vi "Database.GetThisStatus.vi"(7 "system":string, 8 "error in":errorcluster, 9 "Serial":string, 10 "Variant":string, 11 "Data in":T1 {"Variant"."TS"."TV"."minimum" format="%#.3f"; "Variant"."TS"."TV"."maximum" format="%#.3f"; "Variant"."TS"."TP"."value" format="%#.3f"}) -> (0 "error out":errorcluster, 1 "Repetitions":u8, 2 "Status":i8, 3 "Data out":T1 {"Variant"."TS"."TV"."minimum" format="%#.3f"; "Variant"."TS"."TV"."maximum" format="%#.3f"; "Variant"."TS"."TP"."value" format="%#.3f"})   [LabVIEW 2016]
uses:
  Database.Main.Data.ctl
  Database.Main.Data.Status.ctl
  Database.Main.Data.Sets.ctl
  Database.Main.Data.Results.ctl
  ProdaNG/Controls/ProdaNG.Identification.ctl
  ProdaNG/Controls/ProdaNG.ProcessResult.ctl
  ProdaNG/Controls/ProdaNG.ProcessStepResult.ctl
  ProdaNG/Controls/ProdaNG.TestStepResult.ctl
  ProdaNG/Controls/ProdaNG.TestValueResult.ctl
  Database.Main.Data.Variant.ctl
  ProdaNG/Controls/ProdaNG.ProcessStepParam.ctl
  ProdaNG/Controls/ProdaNG.TestStep.ctl
  ProdaNG/Controls/ProdaNG.TestStepParam.ctl
  ProdaNG/Controls/ProdaNG.TestValue.ctl
  tools/EventLog/EventLog.EventLevel.ctl
  tools/EventLog/EventLog.EventSource.ctl
  tools/Translator/Translator.Message.ctl
  tools/EventLog/EventLog.New(array).vi
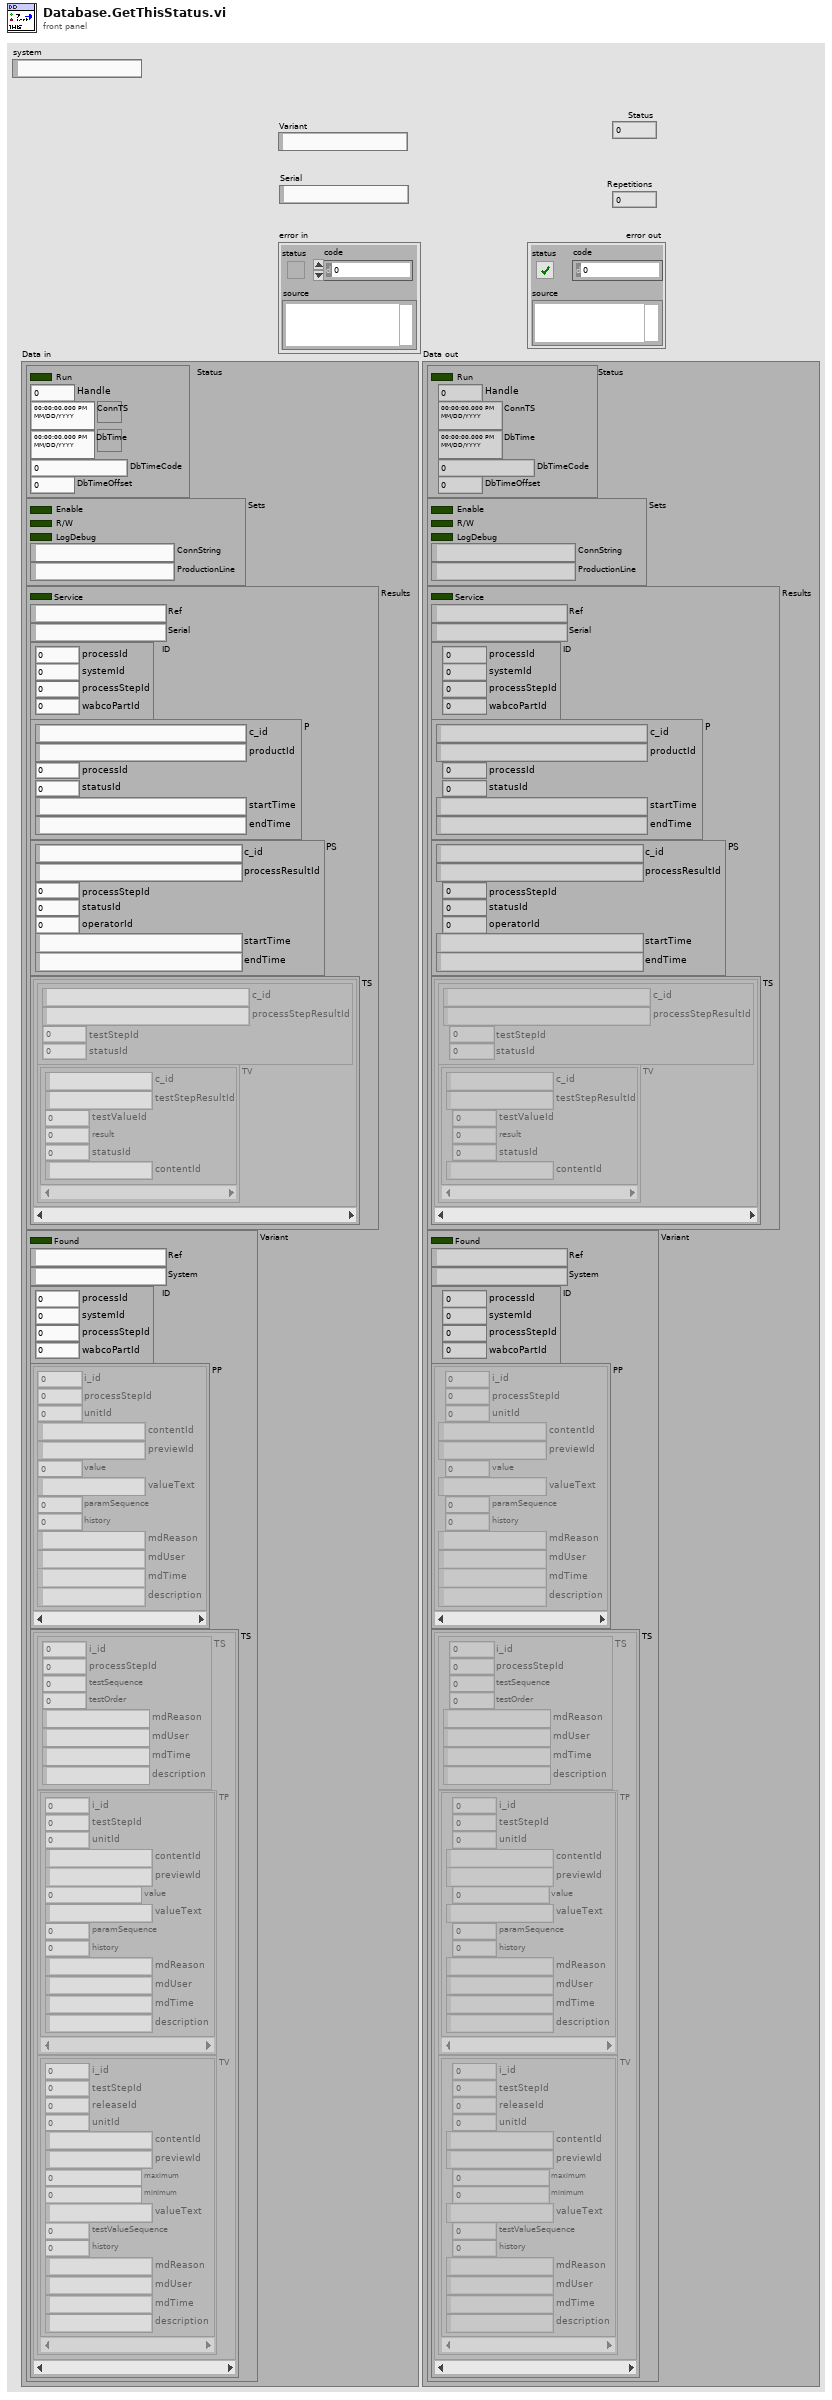
[diagram p1: front panel]
types:
  T1 = typedef "Database.Main.Data.ctl" = cluster{"Status":T2, "Sets":T3, "Results":T4, "Variant":T10}
  T2 = typedef "Database.Main.Data.Status.ctl" = cluster{"Run":bool, "Handle":i32, "ConnTS":timestamp, "DbTime":timestamp, "DbTimeCode":dbl, "DbTimeOffset":dbl}
  T3 = typedef "Database.Main.Data.Sets.ctl" = cluster{"Enable":bool, "R/W":bool, "LogDebug":bool, "ConnString":string, "ProductionLine":string}
  T4 = typedef "Database.Main.Data.Results.ctl" = cluster{"Service":bool, "Ref":string, "Serial":string, "ID":T5, "P":T6, "PS":T7, "TS":cluster{"TS":T8, "TV":T9[]}[]}
  T5 = typedef "ProdaNG.Identification.ctl" = cluster{"processId":i32, "systemId":i32, "processStepId":i32, "wabcoPartId":i32}
  T6 = typedef "ProdaNG.ProcessResult.ctl" = cluster{"c_id":string, "productId":string, "processId":i32, "statusId":i32, "startTime":string, "endTime":string}
  T7 = typedef "ProdaNG.ProcessStepResult.ctl" = cluster{"c_id":string, "processResultId":string, "processStepId":i32, "statusId":i32, "operatorId":i32, "startTime":string, "endTime":string}
  T8 = typedef "ProdaNG.TestStepResult.ctl" = cluster{"c_id":string, "processStepResultId":string, "testStepId":i32, "statusId":i32}
  T9 = typedef "ProdaNG.TestValueResult.ctl" = cluster{"c_id":string, "testStepResultId":string, "testValueId":i32, "result":dbl, "statusId":i32, "contentId":string}
  T10 = typedef "Database.Main.Data.Variant.ctl" = cluster{"Found":bool, "Ref":string, "System":string, "ID":T5, "PP":T11[], "TS":cluster{"TS":T12, "TP":T13[], "TV":T14[]}[]}
  T11 = typedef "ProdaNG.ProcessStepParam.ctl" = cluster{"i_id":i32, "processStepId":i32, "unitId":i32, "contentId":string, "previewId":string, "value":dbl, "valueText":string, "paramSequence":i32, "history":i32, "mdReason":string, "mdUser":string, "mdTime":string, "description":string}
  T12 = typedef "ProdaNG.TestStep.ctl" = cluster{"i_id":i32, "processStepId":i32, "testSequence":i32, "testOrder":i32, "mdReason":string, "mdUser":string, "mdTime":string, "description":string}
  T13 = typedef "ProdaNG.TestStepParam.ctl" = cluster{"i_id":i32, "testStepId":i32, "unitId":i32, "contentId":string, "previewId":string, "value":dbl, "valueText":string, "paramSequence":i32, "history":i32, "mdReason":string, "mdUser":string, "mdTime":string, "description":string}
  T14 = typedef "ProdaNG.TestValue.ctl" = cluster{"i_id":i32, "testStepId":i32, "releaseId":i32, "unitId":i32, "contentId":string, "previewId":string, "maximum":dbl, "minimum":dbl, "valueText":string, "testValueSequence":i32, "history":i32, "mdReason":string, "mdUser":string, "mdTime":string, "description":string}
  T15 = typedef "Translator.Message.ctl" = enum16{"-", "Event confirmed", "Log out", "Log in", "Shutdown", "Cancel", "Start", "Begin time", "End time", "Duration", "Service Mode", "Ignore Results", "Serial Format", "On", "Off", "OK", "NOK", "NOK %s", "Home", "Work", "Close", "Open", "In progress...", "Missing", "Empty", "Hardware failure", "Initial", "Default", "Total", "Out of range", "Free disk space is below 1GB - contact technician", "Error %d >> %s", "Error %d >> %s >> %s", "Msg %d >> %s", "Laser msg %d %s", "Laser cmd error %s %d", "Laser cmd failed %s", "Laser cmd warning %s", "Laser disconnected", "Laser status %s", "Laser already started", "Laser job unkonwn %s", "Laser job missing %s", "Laser job select failure %s", "Unable to start laser printing (%s)", "Unable to stop laser printing (%s)", "Laser marking aborted", "Laser marking timeout", "Unable to reset Laser Interlock (%s)", "Unable to trigger Laser. Laser not ready (%s)", "Laser job '%s' coordinates not configured", "Starting %s", "Quitting %s", "Configured", "Initializing", "Quitting", "Loading", "Loaded %d results", "Loaded %d events", "Running", "Stopped", "Summary", "Laser", "Do you want to continue?", "Do you want to delete the configuration?", "The configuration is being used by an order. Unable to delete!", "Press confirm button", "Station is not based. Do you want to exit?", "Station requires changeover. Do you want to run the test?", "Test options are not set as default. Do you want to continue?", "Formatting of WabcoNo is disabled. Do you want to continue?", "Product not detected. Do you want to continue?", "Product scan failed. Do you want to continue?", "Calibration", "Log out?", "System", "All", "IDLE", "Translating...%s", "Not found", "Alarm %s", "Run", "Skip", "Abort", "Repeat", "Please wait...", "Database disconnected", "Database disconnected - changeover disabled!", "Login to database successful", "Login to database failed: %d; %s", "Unable to check the product status of reference %d - database disconnected", "Unable to set the product status of reference %d - database disconnected", "Variant file backup %s", "Read variant (%s)", "Result", "Station armed!", "Station requires changeover!", "Select reference number...", "EMERGENCY BUTTON - press Control button", "EMERGENCY DOOR - press Control button", "Resetting Emergency...", "Unable to reset safety circuit - Emergency Button pressed", "Unable to reset safety circuit - Emergency Side Door open", "Station not based", "Station based", "Station not empty", "Station basing...", "No order", "Press Start to begin new order", "Scanning new order", "Order NOK. Correct or scan again", "Order OK. Press Accept", "Order ready", "Revolver incorrect", "Fork incorrect", "Revolver missing", "Revolver empty", "Container missing", "Offline results", "Offline statistics", "Updating statistics %.1f %%", "DMC Configurator", "Door open", "Close the front door", "Press start button", "Done. Open the front door", "Running...", "Running...%.1f %%", "Pause %s", "Pause %s. NOK container missing", "Pause %s. OK container missing", "Pause %s. Revolver empty", "Pause %s. Revolver missing", "Pause %s. Revolver incorrect", "Pause %s. Fork missing", "Pause %s. Fork incorrect", "Pause %s. Too many failures", "Pause %s. Unloading failure", "Pause %s. One slot is not working", "Pause %s. Part order is done. Empty OK container", "Pause %s. Unable to move product to slot", "Pause %s. Unable to move back product pusher", "Pause %s. Unable to lift product", "Pause %s. Unable to move back product lifter", "Pause %s. Unable to move product arm to Work", "Pause %s. Unable to move product arm to NOK", "Pause %s. Unable to move product arm to OK", "Pause %s. Unable to unsuck the NOK product", "Pause %s. Unable to drop the NOK product", "Pause %s. Product OK missing", "Pause %s. Unable to unsuck the OK product", "Pause %s. Unable to drop the OK product", "Stopping...", "File '%s' is missing", "File '%s' is broken", "File '%s' is running", "Log file started (%s)", "Log file ended (%s)", "Log file stopped (%s)", "Log file ignored (%s)", "Log file exported (%s)", "Log file export failed (%s)", "Wrong serial number in log file", "Wrong reference number in log file", "Test steps are missing", "%s = %.3f", "Process param '%s' not found in DB", "Process param '%s' wrong order", "Process param '%s' value %.3f out of limits (%.3f; %.3f)", "Step%d param '%s' not found in DB", "Step%d param '%s' wrong order", "Step%d param '%s' value %.3f out of limits (%.3f; %.3f)", "Step%d EV '%s' not found in DB", "Step%d EV '%s' wrong order", "\"%s\" not found in DB", "\"%s\" wrong order", "\"%s\" value %.3f out of limits (%.3f; %.3f)", "\"%s\" not found in software", "Process init (%s)", "Process started", "Process restarted", "Process run", "Process done", "Process done - remove OK container", "Process aborted", "Process aborted at work", "Process aborted at home", "Process error", "Process error at home", "Process error at work", "Process close", "Process pause", "Process continue", "Process door open", "Process door close", "Process pause at slot %s due to %s", "Select plate from the order to process", "Do you want to start the process?", "Do you want to continue the process?", "There is unfinished order. Do you want to put the new order?", "Product %s %d OK", "Product %s %d NOK", "Unable to unload the slot %s. Product missing in the slot", "Unable to unload the slot %s. Product already in the arm", "Unable to accept the product as OK. Product missing in slot %s", "Unable to accept the product as OK. Product could not drop into the container at slot %s", "Unable to accept the product as NOK. Product could not drop into the container at slot %s", "Scan failed. Error %s", "Scan failed. Scanner disconnected", "Scan failed. Wrong Wabco number %d, limit (%d,%d)", "Scan failed. Wrong serial number %d, limit (%d,%d)", "Scan failed. Wrong date %d, limit (%d,%d)", "Scan failed. Wrong product wabco number %d (expected %d)", "Scan failed. Wrong product serial number %d (expected > 0)", "Scan OK %s", "Scan failed. Unable to determine table position (%s)", "Scan failed. Timeout", "Tune failed. Scanner disconnected", "Tune failed. Timeout", "%s = %d", "%s = %d->%d", "Unable to set %s = %.2f - Air Pressure Inside off", "Unable to set digital output '%s' = %d", "Unable to activate air pressure inside - timeout", "Unable to activate air pressure inside - aborted", "Unable to switch on Air Main Valve - Air Pressure Inlet off", "Unable to switch on Air Main Valve - Door open", "Unable to switch off Air Main Valve - timeout", "Unable to switch off Air Main Valve - aborted", "Unable to rotate Table - timeout", "Unable to rotate Table - aborted", "Unable to rotate Table - Product Move not in Home position", "Unable to rotate Table - Air Pressure Inside off", "Unable to rotate Table - Product Lift A not in Home position", "Unable to rotate Table - Product Lift B not in Home position", "Unable to rotate Table - unlock before movement timeout", "Unable to rotate Table - lock after movement timeout", "Unable to move Table Lock to %s position - timeout", "Unable to move Table Lock to %s position - aborted", "Unable to move Table Lock to %s position - Air Pressure Inside off", "Unable to move Table Lock to %s position - Table not in position", "Unable to move Product Lift A to %s position - timeout", "Unable to move Product Lift B to %s position - timeout", "Unable to move Product Lift A to %s position - aborted", "Unable to move Product Lift B to %s position - aborted", "Unable to move Product Lift A to %s position - Air Pressure Inside off", "Unable to move Product Lift B to %s position - Air Pressure Inside off", "Unable to move Product Lift A to %s position - Table not locked", "Unable to move Product Lift B to %s position - Table not locked", "Unable to move Product Lift A to %s position - Product Arm not in Work position", "Unable to move Product Lift B to %s position - Product Arm not in Work position", "Unable to set Product Suction Gripper %s to %s - timeout", "Unable to set Product Suction Gripper %s to %s - aborted", "Unable to set Product Suction Gripper %s to %s - Air Pressure Inside off", "Unable to set Product Suction Gripper %s to %s - Table slot unkown", "Unable to move Product Arm to %s position - timeout", "Unable to move Product Arm to %s position - aborted", "Unable to move Product Arm to %s position - Air Pressure Inside off", "Unable to move Product Arm to %s position - Product Lift A not in Home position", "Unable to move Product Arm to %s position - Product Lift B not in Home position", "Unable to move Product to %s position - timeout", "Unable to move Product to %s position - aborted", "Unable to move Product to %s position - Air Pressure Inside off", "Unable to move Product to %s position - Table not in position"}
  T16 = typedef "EventLog.EventSource.ctl" = enum16{"All", "Gui", "Ref", "File", "Arch", "Seq", "CPX", "DB", "Laser", "Scan.P", "Scan.O", "PLC"}
  T17 = typedef "EventLog.EventLevel.ctl" = enum8{"Debug", "Info", "Warning", "Error"}
  T18 = typedef "ProdaNG.Product.ctl" = cluster{"c_id":string, "wabcoPartId":i32, "serialNumber":string, "comment":string, "individual":i32, "crProcessStepId":i32, "mdProcessStepId":i32, "crTime":string, "mdTime":string}
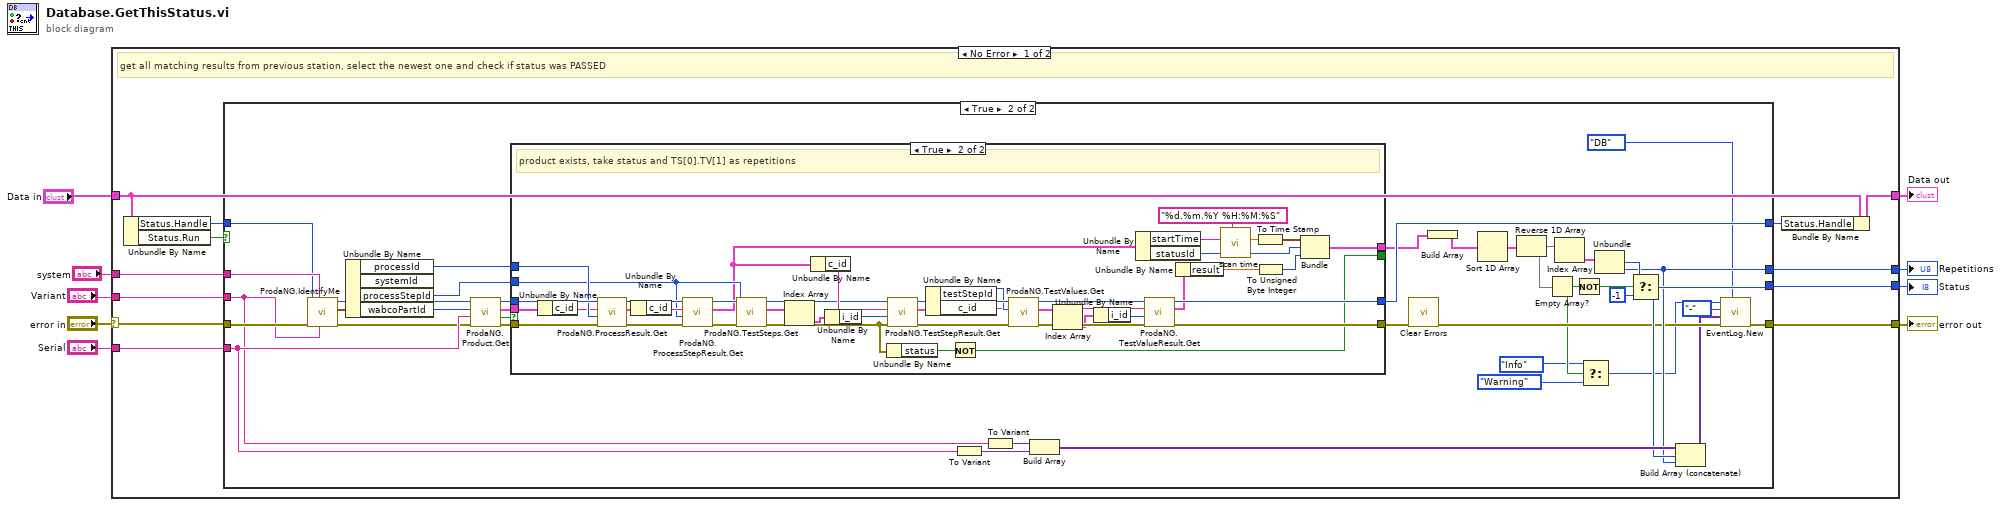
[diagram p0: block diagram]
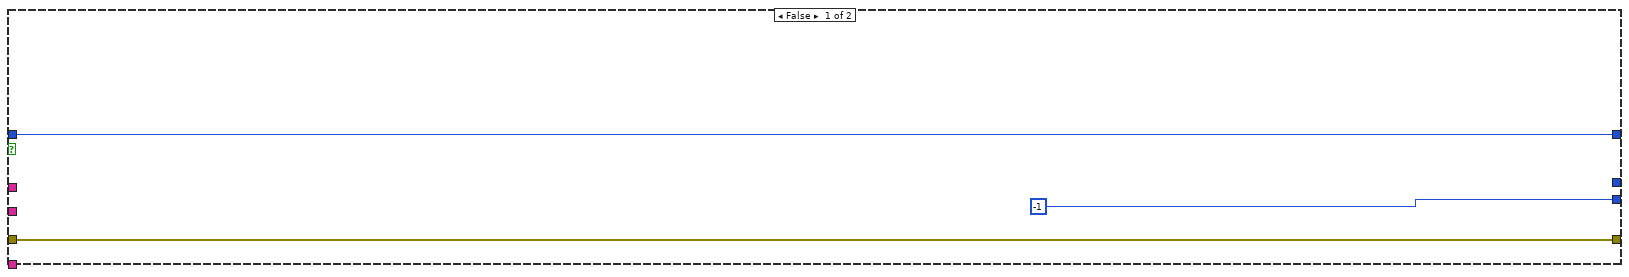
[diagram p2: hidden frame]
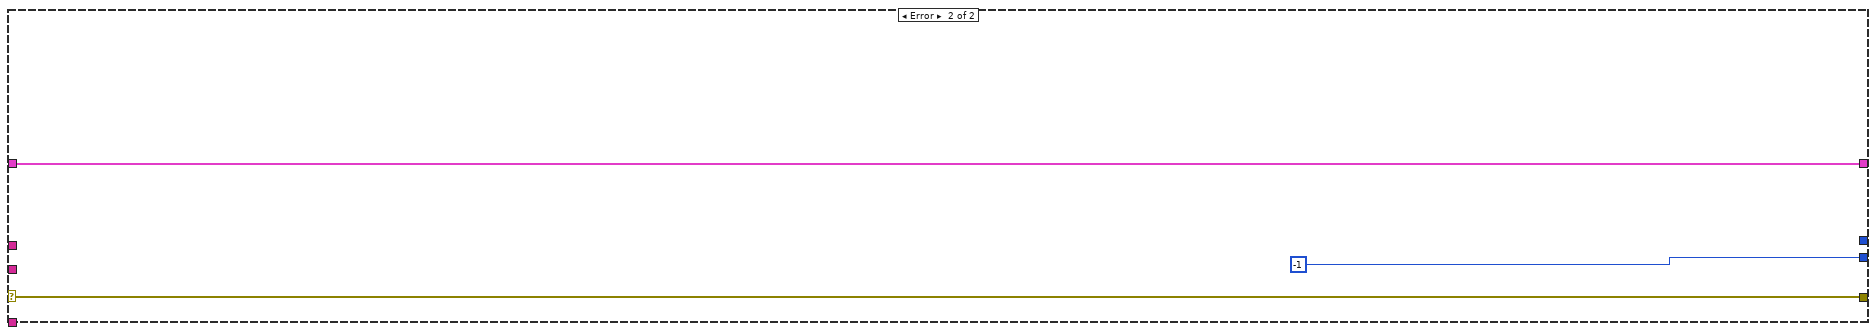
[diagram p4: hidden frame]
diagram:
  n1 = case shown="No Error" "error in" {
    selector: "error in" -> [w20 w110]
    tunnel: [w21 w110] -> w9
    tunnel: "Data in" -> [w18 w109]
    tunnel: [w17 w109] -> w1
    tunnel: "Serial" -> [w14 _]
    tunnel: "Variant" -> [w13 _]
    tunnel: [w12 -1 ("f")] -> w5
    tunnel: [w11 _] -> w4
    tunnel: "system" -> [w10 _]
    frame No Error {
      # "get all matching results from previous station, select the newest one and check if status was PASSED"
      n2 = Unbundle By Name(w18) -> ("Status.Handle"=w19:i32, "Status.Run"=w15:bool)
      n3 = case shown="True" w15 {
        tunnel: w20 -> [w23 w38]
        tunnel: [w23 w49] -> w21
        tunnel: w19 -> [w24 w33]
        tunnel: [w24 w63] -> w16
        tunnel: w14 -> [_ w53]
        tunnel: w13 -> [_ w35]
        tunnel: [-1 ("f") w52] -> w12
        tunnel: [_ w51] -> w11
        tunnel: w10 -> [_ w36]
        frame False {
        }
        frame True {
          n4 = call "ProdaNG.IdentifyMe.vi"("wabcoNumber"=w35, "systemName"=w36, "error in"=w38, "dbHandleIn"=w33) -> ("error out"=w37:errorcluster, "Identification"=w34:T5, "dbHandle"=w32:i32)  [unwired: 5 in]
          n5 = Unbundle By Name(w34) -> ("processId"=w30:i32, "processStepId"=w29:i32, "wabcoPartId"=w31:i32)  [unwired: 1 out]
          n6 = call "ProdaNG.Product.Get.vi"("error in (no error)"=w37, "serialNumber"=w53, "wabcoPartId"=w31, "dbHandle"=w32) -> ("error out"=w41:errorcluster, "found"=w39:bool, "Product"=w40:T18, "dbHandle out"=w42:i32)  [unwired: 4 in]
          n7 = case shown="True" w39 {
            tunnel: w41 -> [w65 w107]
            tunnel: [w65 w89] -> w43
            tunnel: w42 -> [w64 w105]
            tunnel: w40 -> [_ w106]
            tunnel: w29 -> [_ w73]
            tunnel: w30 -> [_ w104]
            tunnel: [_ w84] -> _
            tunnel: [w64 w90] -> w63
            tunnel: [_ w94] -> w28
            frame False {
              # "product missing"
            }
            frame True {
              # "product exists, take status and TS[0].TV[1] as repetitions"
              n8 = Unbundle By Name(w106) -> ("c_id"=w99:string)
              n9 = call "ProdaNG.ProcessResult.Get.vi"("error in (no error)"=w107, "processId"=w104, "productId"=w99, "dbHandle"=w105) -> ("error out"=w101:errorcluster, "ProcessResult"=w103:T6, "dbHandle out"=w102:i32)  [unwired: 4 in, 1 out]
              n10 = Unbundle By Name(w103) -> ("c_id"=w100:string)
              n11 = call "ProdaNG.ProcessStepResult.Get.vi"("error in (no error)"=w101, "processStepId"=w73, "processResultId"=w100, "dbHandle"=w102) -> ("error out"=w72:errorcluster, "ProcessStepResult"=w71:T7, "dbHandle out"=w74:i32)  [unwired: 4 in, 1 out]
              n12 = call "ProdaNG.TestSteps.Get.vi"("error in (no error)"=w72, "processStepId"=w73, "dbHandleIn"=w74) -> ("error out"=w66:errorcluster, "TestSteps"=w69:T12[], "dbHandle"=w70:i32)  [unwired: 6 in]
              n13 = Index Array(array=w69) -> (element=w68:T12)  [unwired: 1 in]
              n14 = Unbundle By Name(w71) -> ("c_id"=w91:string)
              n15 = Unbundle By Name(w68) -> ("i_id"=w67:i32)
              n16 = Unbundle By Name(w66) -> ("status"=w85:bool)
              n17 = call "ProdaNG.TestStepResult.Get.vi"("error in (no error)"=w66, "testStepId"=w67, "processStepResulttId"=w91, "dbHandle"=w70) -> ("error out"=w80:errorcluster, "TestStepResult"=w92:T8, "dbHandle out"=w83:i32)  [unwired: 4 in, 1 out]
              n18 = Unbundle By Name(w92) -> ("testStepId"=w81:i32, "c_id"=w75:string)
              n19 = Not(x=w85) -> (.not. x?=w84:bool)
              n20 = call "ProdaNG.TestValues.Get.vi"("error in (no error)"=w80, "testStepId"=w81, "dbHandleIn"=w83) -> ("error out"=w79:errorcluster, "TestStepValues"=w78:T14[], "dbHandle"=w82:i32)  [unwired: 6 in]
              n21 = Index Array(array=w78) -> (element=w77:T14)  [unwired: 1 in]
              n22 = Unbundle By Name(w77) -> ("i_id"=w76:i32)
              n23 = Unbundle By Name(w71) -> ("startTime"=w96:string, "statusId"=w93:i32)
              n24 = call "ProdaNG.TestValueResult.Get.vi"("error in (no error)"=w79, "testValueId"=w76, "testStepResultId"=w75, "dbHandle"=w82) -> ("error out"=w89:errorcluster, "TestValueResult"=w88:T9, "dbHandle"=w90:i32)  [unwired: 5 in]
              n25 = Unbundle By Name(w88) -> ("result"=w87:dbl)
              n26 = call "scan time.vi"("time format string"="%d.%m.%Y %H:%M:%S", "formatted time string"=w96) -> ("lv time (UTC)"=w97:dbl)  [unwired: 5 in, 4 out]
              n27 = To Time Stamp(1:w97) -> (0:w95:timestamp)
              n28 = To Unsigned Byte Integer(number=w87) -> (unsigned 8bit integer=w86:u8)
              n29 = Bundle(w95, "statusId"=w93, w86) -> (w94:cluster{timestamp, "statusId":i32, u8})  [unwired: 1 in]
            }
          }
          n30 = To Variant(anything=w53) -> (Variant=w55:variant)
          n31 = To Variant(anything=w35) -> (Variant=w56:variant)
          n32 = Build Array(w56, w55) -> (w54:variant[])
          n33 = call <vilib>:"Clear Errors.vi"("error in (no error)"=w43) -> ("error out"=w50:errorcluster)  [unwired: 5 in, 1 out]
          n34 = Build Array(w28) -> (w27:cluster{timestamp, "statusId":i32, u8}[])
          n35 = Sort 1D Array(array=w27) -> (sorted array=w62:cluster{timestamp, "statusId":i32, u8}[])
          n36 = Reverse 1D Array(array=w62) -> (reversed array=w60:cluster{timestamp, "statusId":i32, u8}[])
          n37 = Empty Array?(array=w60) -> (empty?=w47:bool)
          n38 = Index Array(array=w60) -> (element=w61:cluster{timestamp, "statusId":i32, u8})  [unwired: 1 in]
          n39 = Not(x=w47) -> (.not. x?=w59:bool)
          n40 = Select(t=EventLog.EventLevel."Info" ("Level (Info)"), s=w47, f=EventLog.EventLevel."Warning" ("Level (Info)")) -> (s? t:f=w44:T17)
          n41 = Unbundle(w61) -> ("statusId"=w58:i32, w51:u8)  [unwired: 1 out]
          n42 = Select(t=w58, s=w59, f=-1) -> (s? t:f=w52:i32)
          n43 = Build Array (concatenate)(w54, w52, w51) -> (w48:variant[])
          n44 = call-poly "EventLog.New.vi"("Source (All)"=EventLog.EventSource."DB" ("Event source"), "error in (no error)"=w50, "Arguments"=w48, "Message (-)"=Translator.Message."-", "Level (Info)"=w44) -> ("error out"=w49:errorcluster)  [unwired: 5 in, 1 out]
        }
      }
      n45 = Bundle By Name(cluster=w18, "Status.Handle"=w16) -> (w17:T1)
    }
    frame Error {
    }
  }
  "error out" <- w9
  "Status" <- w5
  "Repetitions" <- w4
  "Data out" <- w1
